vi "Format SN PN.vi"(0 "Barcode":string, 11 "Error In":errorcluster) -> (4 "Part":string, 8 "Serial":string, 15 "Error Out":errorcluster)   [LabVIEW 2021]
doc: "Takes in a barcode similar to P:10-06104CR:03S:SIE251201167 and returns a part number and serial number pair as the IPC expects: 1006104C03 and SIE251201167."
uses:
  <vilib>/regexp/Match Regular Expression.xnode
panel:
  # "Inputs"
  # "Outputs"
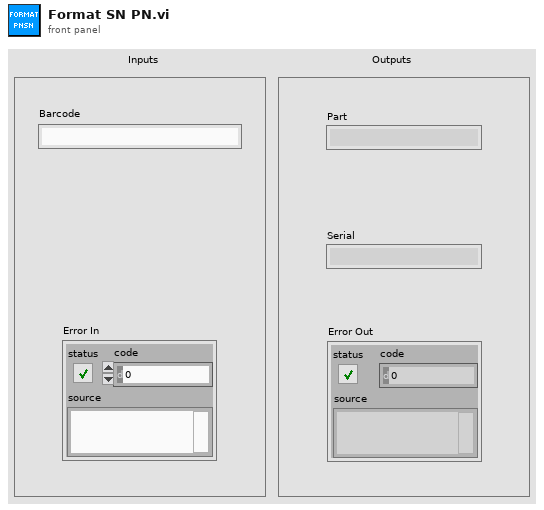
[diagram p1: front panel]
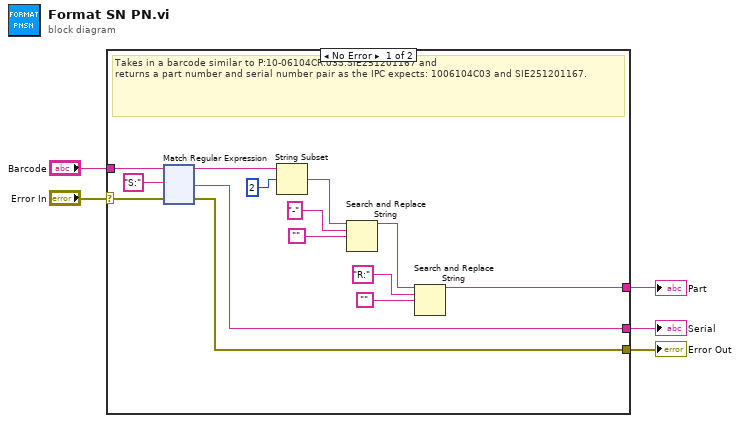
[diagram p0: block diagram]
diagram:
  n1 = case shown="No Error" "Error In" {
    selector: "Error In" -> [w17 w137]
    tunnel: "Barcode" -> [w19 _]
    tunnel: [w12 w137] -> w3
    tunnel: [w13 _] -> w2
    tunnel: [w6 _] -> w1
    frame No Error {
      # "Takes in a barcode similar to P:10-06104CR:03S:SIE251201167 and \nreturns a part number and serial number pair as the IPC expects: 1006104C03 and SIE251201167."
      n2 = xnode "Match Regular Expression"("input string"=w19, "regular expression"="S:", "error in"=w17) -> ("before match"=w16:string, "after match"=w13:string, "error out"=w12:errorcluster)  [unwired: 3 in, 2 out]
      n3 = String Subset(string=w16, offset (0)=2) -> (substring=w14:string)  [unwired: 1 in]
      n4 = Search and Replace String(input string=w14, search string="-", replace string="") -> (result string=w8:string)  [unwired: 5 in, 3 out]
      n5 = Search and Replace String(input string=w8, search string="R:", replace string="") -> (result string=w6:string)  [unwired: 5 in, 3 out]
    }
    frame Error {
      # "Can't start due to error"
    }
  }
  "Error Out" <- w3
  "Serial" <- w2
  "Part" <- w1
